vi "main(Test DQMH modules).vi"() -> ()   [LabVIEW 2018, in "Application.lvlib"] (continued)
                n6100 = To Variant(anything=T3."mux10_1_channel6" ("mux10_1(x6)_encode")) -> (Variant=w13208:variant)
                n6101 = To Variant(anything=T4."demux1_10_channel6" ("demux1_10(x6)_encode")) -> (Variant=w13204:variant)
                n6102 = To Variant(anything=bool[] [FALSE, FALSE, FALSE, TRUE, FALSE, FALSE]) -> (Variant=w13219:variant)
                n6103 = Bundle By Name(cluster=w13210, "command"="MEAS.AllRelaysOFF") -> (w13218:T9)
                n6104 = Bundle By Name(cluster=w13210, "command"="MEAS.mux10-1", "data"=w13208) -> (w13201:T9)
                n6105 = Bundle By Name(cluster=w13210, "command"="MEAS.demux1-10", "data"=w13204) -> (w13202:T9)
                n6106 = Bundle By Name(cluster=w13210, "command"="MEAS.eMIC", "data"=w13219) -> (w13203:T9)
                n6107 = Build Array(w13218, w13201, w13202, w13203) -> (w13196:T9[])
                n6108 = To Variant(anything=w13200) -> (Variant=w13199:variant)
                n6109 = To Variant(anything=w13200) -> (Variant=w13198:variant)
                n6110 = Bundle By Name(cluster=w13197, "command"="MEAS.requestAC", "data"=w13199) -> (w13216:T9)
                n6111 = Bundle By Name(cluster=w13197, "command"="Apps.WaitForEvent", "data"=w13198) -> (w13212:T9)
                n6112 = Bundle By Name(cluster=w13197, "command"="Apps.UI Update 1") -> (w13213:T9)
                n6113 = Bundle By Name(cluster=w13197, "command"="WaitFor") -> (w13195:T9)
                n6114 = Build Array (concatenate)(w13196, w13195, w13216, w13212, w13213) -> (w13211:T9[])
              }
              frame True {
                w13226 = T9 {"command"="", "data"=variant} ("element")
                w13248 = T9 {"command"="", "data"=variant} ("element")
                n6115 = To Variant(anything=T3."mux10_1_channel6" ("mux10_1(x6)_encode")) -> (Variant=w13255:variant)
                n6116 = To Variant(anything=T2."mux6_1_channel4_3" ("mux6_1(3wires)_encode")) -> (Variant=w13253:variant)
                n6117 = To Variant(anything=T4."demux1_10_channel6" ("demux1_10(x6)_encode")) -> (Variant=w13249:variant)
                n6118 = To Variant(anything=bool[] [FALSE, FALSE, FALSE, TRUE, FALSE, FALSE]) -> (Variant=w13245:variant)
                n6119 = Bundle By Name(cluster=w13248, "command"="MEAS.AllRelaysOFF") -> (w13244:T9)
                n6120 = Bundle By Name(cluster=w13248, "command"="MEAS.mux10-1", "data"=w13255) -> (w13243:T9)
                n6121 = Bundle By Name(cluster=w13248, "command"="MEAS.mux6_1", "data"=w13253) -> (w13242:T9)
                n6122 = Bundle By Name(cluster=w13248, "command"="MEAS.demux1-10", "data"=w13249) -> (w13241:T9)
                n6123 = Bundle By Name(cluster=w13248, "command"="MEAS.eMIC", "data"=w13245) -> (w13240:T9)
                n6124 = Build Array(w13244, w13243, w13242, w13241, w13240) -> (w13225:T9[])
                n6125 = To Variant(anything=w13230) -> (Variant=w13228:variant)
                n6126 = To Variant(anything=w13230) -> (Variant=w13227:variant)
                n6127 = Bundle By Name(cluster=w13226, "command"="WaitFor") -> (w13224:T9)
                n6128 = Bundle By Name(cluster=w13226, "command"="MEAS.DMM dual read") -> (w13237:T9)
                n6129 = Bundle By Name(cluster=w13226, "command"="MEAS.requestAC", "data"=w13228) -> (w13236:T9)
                n6130 = Bundle By Name(cluster=w13226, "command"="Apps.WaitForEvent", "data"=w13227) -> (w13231:T9)
                n6131 = Bundle By Name(cluster=w13226, "command"="Apps.UI Update 1") -> (w13232:T9)
                n6132 = Build Array (concatenate)(w13225, w13224, w13237, w13236, w13231, w13232) -> (w13229:T9[])
              }
            }
          }
          frame True {
            n6133 = Bundle By Name(cluster=T9 {"command"="", "data"=variant} ("element"), "command"="Apps.UI Update 1") -> (w13259:T9)
            n6134 = Build Array(w13259) -> (w13258:T9[])
          }
        }
        n6135 = for {
          tunnel: w13174 -> [w13269] mode=indexing
          tunnel: w13182 -> [w13270]
          tunnel: [w13266] -> w13184 mode=indexing
          n6136 = Unbundle By Name(w13269) -> ("command"=w13268:string, "data"=w13267:variant)
          n6137 = call "App enquece.vi"("command data"=w13267, "command"=w13268, "queue in"=w13270) -> ("error out"=w13266:errorcluster)  [unwired: 7 in, 1 out]
        }
        n6138 = Merge Errors(w13185, w13184) -> (w13183:errorcluster)
      }
      frame "Test DRV 35A" {
        w13274 = 35 ("DUT index(0-59)")
        n6139 = disable-structure shown="LOGGING==TRUE" {
          disable-tunnel: w13279 -> [w13362 _]
          frame condition #0 (active) {
            n6140 = Empty String/Path?(string/path=w13362) -> (empty?=w13364:bool)
            n6141 = Select(t="Quece timeout", s=w13364, f=w13362) -> (s? t:f=w13361:string)
            n6142 = call "string log (SubVI).vi"("state Name"=w13361) -> ()  [unwired: 9 in, 2 out]
          }
          frame condition #1 {
          }
        }
        n6143 = Flush Queue(queue=w13280) -> (queue out=w13281:refnum<queue>)  [unwired: 1 in, 2 out]
        n6144 = Decrement(x=w13274) -> (x-1=w13278:i32)
        n6145 = Index Array(array=w13275, index=w13278) -> (element=w13276:refnum<vi>)
        n6146 = call "FGV DRV stand.vi"() -> ("Sub-Test.DCV"=w13271:bool)  [unwired: 10 in, 1 out]
        n6147 = call "FGV Driver Data.vi"("DUT index(1-60)"=w13274) -> ("DUT SC"=w13272:bool)  [unwired: 7 in, 3 out]
        n6148 = property class="ColBox"(reference=w13276, "Value"=u32 10000536 ("DRV 1")) -> ()  [unwired: 1 in, 2 out]
        n6149 = case shown="False" w13272 {
          tunnel: w13274 -> [w13292 _]
          tunnel: [w13291 w13357] -> w13273
          tunnel: w13271 -> [w13290 _]
          frame False {
            n6150 = case shown="True" w13290 {
              tunnel: w13292 -> [w13299 w13329]
              tunnel: [w13310 w13328] -> w13291
              frame False {
                w13296 = T9 {"command"="", "data"=variant} ("element")
                w13309 = T9 {"command"="", "data"=variant} ("element")
                n6151 = To Variant(anything=T3."mux10_1_channel6" ("mux10_1(x6)_encode")) -> (Variant=w13307:variant)
                n6152 = To Variant(anything=T4."demux1_10_channel6" ("demux1_10(x6)_encode")) -> (Variant=w13303:variant)
                n6153 = To Variant(anything=bool[] [FALSE, FALSE, FALSE, FALSE, TRUE, FALSE]) -> (Variant=w13318:variant)
                n6154 = Bundle By Name(cluster=w13309, "command"="MEAS.AllRelaysOFF") -> (w13317:T9)
                n6155 = Bundle By Name(cluster=w13309, "command"="MEAS.mux10-1", "data"=w13307) -> (w13300:T9)
                n6156 = Bundle By Name(cluster=w13309, "command"="MEAS.demux1-10", "data"=w13303) -> (w13301:T9)
                n6157 = Bundle By Name(cluster=w13309, "command"="MEAS.eMIC", "data"=w13318) -> (w13302:T9)
                n6158 = Build Array(w13317, w13300, w13301, w13302) -> (w13295:T9[])
                n6159 = To Variant(anything=w13299) -> (Variant=w13298:variant)
                n6160 = To Variant(anything=w13299) -> (Variant=w13297:variant)
                n6161 = Bundle By Name(cluster=w13296, "command"="MEAS.requestAC", "data"=w13298) -> (w13315:T9)
                n6162 = Bundle By Name(cluster=w13296, "command"="Apps.WaitForEvent", "data"=w13297) -> (w13311:T9)
                n6163 = Bundle By Name(cluster=w13296, "command"="Apps.UI Update 1") -> (w13312:T9)
                n6164 = Bundle By Name(cluster=w13296, "command"="WaitFor") -> (w13294:T9)
                n6165 = Build Array (concatenate)(w13295, w13294, w13315, w13311, w13312) -> (w13310:T9[])
              }
              frame True {
                w13325 = T9 {"command"="", "data"=variant} ("element")
                w13347 = T9 {"command"="", "data"=variant} ("element")
                n6166 = To Variant(anything=T3."mux10_1_channel6" ("mux10_1(x6)_encode")) -> (Variant=w13354:variant)
                n6167 = To Variant(anything=T2."mux6_1_channel5_3" ("mux6_1(3wires)_encode")) -> (Variant=w13352:variant)
                n6168 = To Variant(anything=T4."demux1_10_channel6" ("demux1_10(x6)_encode")) -> (Variant=w13348:variant)
                n6169 = To Variant(anything=bool[] [FALSE, FALSE, FALSE, FALSE, TRUE, FALSE]) -> (Variant=w13344:variant)
                n6170 = Bundle By Name(cluster=w13347, "command"="MEAS.AllRelaysOFF") -> (w13343:T9)
                n6171 = Bundle By Name(cluster=w13347, "command"="MEAS.mux10-1", "data"=w13354) -> (w13342:T9)
                n6172 = Bundle By Name(cluster=w13347, "command"="MEAS.mux6_1", "data"=w13352) -> (w13341:T9)
                n6173 = Bundle By Name(cluster=w13347, "command"="MEAS.demux1-10", "data"=w13348) -> (w13340:T9)
                n6174 = Bundle By Name(cluster=w13347, "command"="MEAS.eMIC", "data"=w13344) -> (w13339:T9)
                n6175 = Build Array(w13343, w13342, w13341, w13340, w13339) -> (w13324:T9[])
                n6176 = To Variant(anything=w13329) -> (Variant=w13327:variant)
                n6177 = To Variant(anything=w13329) -> (Variant=w13326:variant)
                n6178 = Bundle By Name(cluster=w13325, "command"="WaitFor") -> (w13323:T9)
                n6179 = Bundle By Name(cluster=w13325, "command"="MEAS.DMM dual read") -> (w13336:T9)
                n6180 = Bundle By Name(cluster=w13325, "command"="MEAS.requestAC", "data"=w13327) -> (w13335:T9)
                n6181 = Bundle By Name(cluster=w13325, "command"="Apps.WaitForEvent", "data"=w13326) -> (w13330:T9)
                n6182 = Bundle By Name(cluster=w13325, "command"="Apps.UI Update 1") -> (w13331:T9)
                n6183 = Build Array (concatenate)(w13324, w13323, w13336, w13335, w13330, w13331) -> (w13328:T9[])
              }
            }
          }
          frame True {
            n6184 = Bundle By Name(cluster=T9 {"command"="", "data"=variant} ("element"), "command"="Apps.UI Update 1") -> (w13358:T9)
            n6185 = Build Array(w13358) -> (w13357:T9[])
          }
        }
        n6186 = for {
          tunnel: w13273 -> [w13368] mode=indexing
          tunnel: w13281 -> [w13369]
          tunnel: [w13365] -> w13283 mode=indexing
          n6187 = Unbundle By Name(w13368) -> ("command"=w13367:string, "data"=w13366:variant)
          n6188 = call "App enquece.vi"("command data"=w13366, "command"=w13367, "queue in"=w13369) -> ("error out"=w13365:errorcluster)  [unwired: 7 in, 1 out]
        }
        n6189 = Merge Errors(w13284, w13283) -> (w13282:errorcluster)
      }
      frame "Test DRV 36A" {
        w13373 = 36 ("DUT index(0-59)")
        n6190 = disable-structure shown="LOGGING==TRUE" {
          disable-tunnel: w13378 -> [w13461 _]
          frame condition #0 (active) {
            n6191 = Empty String/Path?(string/path=w13461) -> (empty?=w13463:bool)
            n6192 = Select(t="Quece timeout", s=w13463, f=w13461) -> (s? t:f=w13460:string)
            n6193 = call "string log (SubVI).vi"("state Name"=w13460) -> ()  [unwired: 9 in, 2 out]
          }
          frame condition #1 {
          }
        }
        n6194 = Flush Queue(queue=w13379) -> (queue out=w13380:refnum<queue>)  [unwired: 1 in, 2 out]
        n6195 = Decrement(x=w13373) -> (x-1=w13377:i32)
        n6196 = Index Array(array=w13374, index=w13377) -> (element=w13375:refnum<vi>)
        n6197 = call "FGV DRV stand.vi"() -> ("Sub-Test.DCV"=w13370:bool)  [unwired: 10 in, 1 out]
        n6198 = call "FGV Driver Data.vi"("DUT index(1-60)"=w13373) -> ("DUT SC"=w13371:bool)  [unwired: 7 in, 3 out]
        n6199 = property class="ColBox"(reference=w13375, "Value"=u32 10000536 ("DRV 1")) -> ()  [unwired: 1 in, 2 out]
        n6200 = case shown="False" w13371 {
          tunnel: w13373 -> [w13391 _]
          tunnel: [w13390 w13456] -> w13372
          tunnel: w13370 -> [w13389 _]
          frame False {
            n6201 = case shown="True" w13389 {
              tunnel: w13391 -> [w13398 w13428]
              tunnel: [w13409 w13427] -> w13390
              frame False {
                w13395 = T9 {"command"="", "data"=variant} ("element")
                w13408 = T9 {"command"="", "data"=variant} ("element")
                n6202 = To Variant(anything=T3."mux10_1_channel6" ("mux10_1(x6)_encode")) -> (Variant=w13406:variant)
                n6203 = To Variant(anything=T4."demux1_10_channel6" ("demux1_10(x6)_encode")) -> (Variant=w13402:variant)
                n6204 = To Variant(anything=bool[] [FALSE, FALSE, FALSE, FALSE, FALSE, TRUE]) -> (Variant=w13417:variant)
                n6205 = Bundle By Name(cluster=w13408, "command"="MEAS.AllRelaysOFF") -> (w13416:T9)
                n6206 = Bundle By Name(cluster=w13408, "command"="MEAS.mux10-1", "data"=w13406) -> (w13399:T9)
                n6207 = Bundle By Name(cluster=w13408, "command"="MEAS.demux1-10", "data"=w13402) -> (w13400:T9)
                n6208 = Bundle By Name(cluster=w13408, "command"="MEAS.eMIC", "data"=w13417) -> (w13401:T9)
                n6209 = Build Array(w13416, w13399, w13400, w13401) -> (w13394:T9[])
                n6210 = To Variant(anything=w13398) -> (Variant=w13397:variant)
                n6211 = To Variant(anything=w13398) -> (Variant=w13396:variant)
                n6212 = Bundle By Name(cluster=w13395, "command"="MEAS.requestAC", "data"=w13397) -> (w13414:T9)
                n6213 = Bundle By Name(cluster=w13395, "command"="Apps.WaitForEvent", "data"=w13396) -> (w13410:T9)
                n6214 = Bundle By Name(cluster=w13395, "command"="Apps.UI Update 1") -> (w13411:T9)
                n6215 = Bundle By Name(cluster=w13395, "command"="WaitFor") -> (w13393:T9)
                n6216 = Build Array (concatenate)(w13394, w13393, w13414, w13410, w13411) -> (w13409:T9[])
              }
              frame True {
                w13424 = T9 {"command"="", "data"=variant} ("element")
                w13446 = T9 {"command"="", "data"=variant} ("element")
                n6217 = To Variant(anything=T3."mux10_1_channel6" ("mux10_1(x6)_encode")) -> (Variant=w13453:variant)
                n6218 = To Variant(anything=T2."mux6_1_channel6_3" ("mux6_1(3wires)_encode")) -> (Variant=w13451:variant)
                n6219 = To Variant(anything=T4."demux1_10_channel6" ("demux1_10(x6)_encode")) -> (Variant=w13447:variant)
                n6220 = To Variant(anything=bool[] [FALSE, FALSE, FALSE, FALSE, FALSE, TRUE]) -> (Variant=w13443:variant)
                n6221 = Bundle By Name(cluster=w13446, "command"="MEAS.AllRelaysOFF") -> (w13442:T9)
                n6222 = Bundle By Name(cluster=w13446, "command"="MEAS.mux10-1", "data"=w13453) -> (w13441:T9)
                n6223 = Bundle By Name(cluster=w13446, "command"="MEAS.mux6_1", "data"=w13451) -> (w13440:T9)
                n6224 = Bundle By Name(cluster=w13446, "command"="MEAS.demux1-10", "data"=w13447) -> (w13439:T9)
                n6225 = Bundle By Name(cluster=w13446, "command"="MEAS.eMIC", "data"=w13443) -> (w13438:T9)
                n6226 = Build Array(w13442, w13441, w13440, w13439, w13438) -> (w13423:T9[])
                n6227 = To Variant(anything=w13428) -> (Variant=w13426:variant)
                n6228 = To Variant(anything=w13428) -> (Variant=w13425:variant)
                n6229 = Bundle By Name(cluster=w13424, "command"="WaitFor") -> (w13422:T9)
                n6230 = Bundle By Name(cluster=w13424, "command"="MEAS.DMM dual read") -> (w13435:T9)
                n6231 = Bundle By Name(cluster=w13424, "command"="MEAS.requestAC", "data"=w13426) -> (w13434:T9)
                n6232 = Bundle By Name(cluster=w13424, "command"="Apps.WaitForEvent", "data"=w13425) -> (w13429:T9)
                n6233 = Bundle By Name(cluster=w13424, "command"="Apps.UI Update 1") -> (w13430:T9)
                n6234 = Build Array (concatenate)(w13423, w13422, w13435, w13434, w13429, w13430) -> (w13427:T9[])
              }
            }
          }
          frame True {
            n6235 = Bundle By Name(cluster=T9 {"command"="", "data"=variant} ("element"), "command"="Apps.UI Update 1") -> (w13457:T9)
            n6236 = Build Array(w13457) -> (w13456:T9[])
          }
        }
        n6237 = for {
          tunnel: w13372 -> [w13467] mode=indexing
          tunnel: w13380 -> [w13468]
          tunnel: [w13464] -> w13382 mode=indexing
          n6238 = Unbundle By Name(w13467) -> ("command"=w13466:string, "data"=w13465:variant)
          n6239 = call "App enquece.vi"("command data"=w13465, "command"=w13466, "queue in"=w13468) -> ("error out"=w13464:errorcluster)  [unwired: 7 in, 1 out]
        }
        n6240 = Merge Errors(w13383, w13382) -> (w13381:errorcluster)
      }
      frame "Test DRV 37A" {
        w13472 = 37 ("DUT index(0-59)")
        n6241 = disable-structure shown="LOGGING==TRUE" {
          disable-tunnel: w13477 -> [w13560 _]
          frame condition #0 (active) {
            n6242 = Empty String/Path?(string/path=w13560) -> (empty?=w13562:bool)
            n6243 = Select(t="Quece timeout", s=w13562, f=w13560) -> (s? t:f=w13559:string)
            n6244 = call "string log (SubVI).vi"("state Name"=w13559) -> ()  [unwired: 9 in, 2 out]
          }
          frame condition #1 {
          }
        }
        n6245 = Flush Queue(queue=w13478) -> (queue out=w13479:refnum<queue>)  [unwired: 1 in, 2 out]
        n6246 = Decrement(x=w13472) -> (x-1=w13476:i32)
        n6247 = Index Array(array=w13473, index=w13476) -> (element=w13474:refnum<vi>)
        n6248 = call "FGV DRV stand.vi"() -> ("Sub-Test.DCV"=w13469:bool)  [unwired: 10 in, 1 out]
        n6249 = call "FGV Driver Data.vi"("DUT index(1-60)"=w13472) -> ("DUT SC"=w13470:bool)  [unwired: 7 in, 3 out]
        n6250 = property class="ColBox"(reference=w13474, "Value"=u32 10000536 ("DRV 1")) -> ()  [unwired: 1 in, 2 out]
        n6251 = case shown="False" w13470 {
          tunnel: w13472 -> [w13490 _]
          tunnel: [w13489 w13555] -> w13471
          tunnel: w13469 -> [w13488 _]
          frame False {
            n6252 = case shown="False" w13488 {
              tunnel: w13490 -> [w13497 w13527]
              tunnel: [w13508 w13526] -> w13489
              frame False {
                w13494 = T9 {"command"="", "data"=variant} ("element")
                w13507 = T9 {"command"="", "data"=variant} ("element")
                n6253 = To Variant(anything=T3."mux10_1_channel7" ("mux10_1(x6)_encode")) -> (Variant=w13505:variant)
                n6254 = To Variant(anything=T4."demux1_10_channel7" ("demux1_10(x6)_encode")) -> (Variant=w13501:variant)
                n6255 = To Variant(anything=bool[] [TRUE, FALSE, FALSE, FALSE, FALSE, FALSE]) -> (Variant=w13516:variant)
                n6256 = Bundle By Name(cluster=w13507, "command"="MEAS.AllRelaysOFF") -> (w13515:T9)
                n6257 = Bundle By Name(cluster=w13507, "command"="MEAS.mux10-1", "data"=w13505) -> (w13498:T9)
                n6258 = Bundle By Name(cluster=w13507, "command"="MEAS.demux1-10", "data"=w13501) -> (w13499:T9)
                n6259 = Bundle By Name(cluster=w13507, "command"="MEAS.eMIC", "data"=w13516) -> (w13500:T9)
                n6260 = Build Array(w13515, w13498, w13499, w13500) -> (w13493:T9[])
                n6261 = To Variant(anything=w13497) -> (Variant=w13496:variant)
                n6262 = To Variant(anything=w13497) -> (Variant=w13495:variant)
                n6263 = Bundle By Name(cluster=w13494, "command"="MEAS.requestAC", "data"=w13496) -> (w13513:T9)
                n6264 = Bundle By Name(cluster=w13494, "command"="Apps.WaitForEvent", "data"=w13495) -> (w13509:T9)
                n6265 = Bundle By Name(cluster=w13494, "command"="Apps.UI Update 1") -> (w13510:T9)
                n6266 = Bundle By Name(cluster=w13494, "command"="WaitFor") -> (w13492:T9)
                n6267 = Build Array (concatenate)(w13493, w13492, w13513, w13509, w13510) -> (w13508:T9[])
              }
              frame True {
                w13523 = T9 {"command"="", "data"=variant} ("element")
                w13545 = T9 {"command"="", "data"=variant} ("element")
                n6268 = To Variant(anything=T3."mux10_1_channel7" ("mux10_1(x6)_encode")) -> (Variant=w13552:variant)
                n6269 = To Variant(anything=T2."mux6_1_channel1_3" ("mux6_1(3wires)_encode")) -> (Variant=w13550:variant)
                n6270 = To Variant(anything=T4."demux1_10_channel7" ("demux1_10(x6)_encode")) -> (Variant=w13546:variant)
                n6271 = To Variant(anything=bool[] [TRUE, FALSE, FALSE, FALSE, FALSE, FALSE]) -> (Variant=w13542:variant)
                n6272 = Bundle By Name(cluster=w13545, "command"="MEAS.AllRelaysOFF") -> (w13541:T9)
                n6273 = Bundle By Name(cluster=w13545, "command"="MEAS.mux10-1", "data"=w13552) -> (w13540:T9)
                n6274 = Bundle By Name(cluster=w13545, "command"="MEAS.mux6_1", "data"=w13550) -> (w13539:T9)
                n6275 = Bundle By Name(cluster=w13545, "command"="MEAS.demux1-10", "data"=w13546) -> (w13538:T9)
                n6276 = Bundle By Name(cluster=w13545, "command"="MEAS.eMIC", "data"=w13542) -> (w13537:T9)
                n6277 = Build Array(w13541, w13540, w13539, w13538, w13537) -> (w13522:T9[])
                n6278 = To Variant(anything=w13527) -> (Variant=w13525:variant)
                n6279 = To Variant(anything=w13527) -> (Variant=w13524:variant)
                n6280 = Bundle By Name(cluster=w13523, "command"="WaitFor") -> (w13521:T9)
                n6281 = Bundle By Name(cluster=w13523, "command"="MEAS.DMM dual read") -> (w13534:T9)
                n6282 = Bundle By Name(cluster=w13523, "command"="MEAS.requestAC", "data"=w13525) -> (w13533:T9)
                n6283 = Bundle By Name(cluster=w13523, "command"="Apps.WaitForEvent", "data"=w13524) -> (w13528:T9)
                n6284 = Bundle By Name(cluster=w13523, "command"="Apps.UI Update 1") -> (w13529:T9)
                n6285 = Build Array (concatenate)(w13522, w13521, w13534, w13533, w13528, w13529) -> (w13526:T9[])
              }
            }
          }
          frame True {
            n6286 = Bundle By Name(cluster=T9 {"command"="", "data"=variant} ("element"), "command"="Apps.UI Update 1") -> (w13556:T9)
            n6287 = Build Array(w13556) -> (w13555:T9[])
          }
        }
        n6288 = for {
          tunnel: w13471 -> [w13566] mode=indexing
          tunnel: w13479 -> [w13567]
          tunnel: [w13563] -> w13481 mode=indexing
          n6289 = Unbundle By Name(w13566) -> ("command"=w13565:string, "data"=w13564:variant)
          n6290 = call "App enquece.vi"("command data"=w13564, "command"=w13565, "queue in"=w13567) -> ("error out"=w13563:errorcluster)  [unwired: 7 in, 1 out]
        }
        n6291 = Merge Errors(w13482, w13481) -> (w13480:errorcluster)
      }
      frame "Test DRV 38A" {
        w13571 = 38 ("DUT index(0-59)")
        n6292 = disable-structure shown="LOGGING==TRUE" {
          disable-tunnel: w13576 -> [w13659 _]
          frame condition #0 (active) {
            n6293 = Empty String/Path?(string/path=w13659) -> (empty?=w13661:bool)
            n6294 = Select(t="Quece timeout", s=w13661, f=w13659) -> (s? t:f=w13658:string)
            n6295 = call "string log (SubVI).vi"("state Name"=w13658) -> ()  [unwired: 9 in, 2 out]
          }
          frame condition #1 {
          }
        }
        n6296 = Flush Queue(queue=w13577) -> (queue out=w13578:refnum<queue>)  [unwired: 1 in, 2 out]
        n6297 = Decrement(x=w13571) -> (x-1=w13575:i32)
        n6298 = Index Array(array=w13572, index=w13575) -> (element=w13573:refnum<vi>)
        n6299 = call "FGV DRV stand.vi"() -> ("Sub-Test.DCV"=w13568:bool)  [unwired: 10 in, 1 out]
        n6300 = call "FGV Driver Data.vi"("DUT index(1-60)"=w13571) -> ("DUT SC"=w13569:bool)  [unwired: 7 in, 3 out]
        n6301 = property class="ColBox"(reference=w13573, "Value"=u32 10000536 ("DRV 1")) -> ()  [unwired: 1 in, 2 out]
        n6302 = case shown="False" w13569 {
          tunnel: w13571 -> [w13589 _]
          tunnel: [w13588 w13654] -> w13570
          tunnel: w13568 -> [w13587 _]
          frame False {
            n6303 = case shown="True" w13587 {
              tunnel: w13589 -> [w13596 w13626]
              tunnel: [w13607 w13625] -> w13588
              frame False {
                w13593 = T9 {"command"="", "data"=variant} ("element")
                w13606 = T9 {"command"="", "data"=variant} ("element")
                n6304 = To Variant(anything=T3."mux10_1_channel7" ("mux10_1(x6)_encode")) -> (Variant=w13604:variant)
                n6305 = To Variant(anything=T4."demux1_10_channel7" ("demux1_10(x6)_encode")) -> (Variant=w13600:variant)
                n6306 = To Variant(anything=bool[] [FALSE, TRUE, FALSE, FALSE, FALSE, FALSE]) -> (Variant=w13615:variant)
                n6307 = Bundle By Name(cluster=w13606, "command"="MEAS.AllRelaysOFF") -> (w13614:T9)
                n6308 = Bundle By Name(cluster=w13606, "command"="MEAS.mux10-1", "data"=w13604) -> (w13597:T9)
                n6309 = Bundle By Name(cluster=w13606, "command"="MEAS.demux1-10", "data"=w13600) -> (w13598:T9)
                n6310 = Bundle By Name(cluster=w13606, "command"="MEAS.eMIC", "data"=w13615) -> (w13599:T9)
                n6311 = Build Array(w13614, w13597, w13598, w13599) -> (w13592:T9[])
                n6312 = To Variant(anything=w13596) -> (Variant=w13595:variant)
                n6313 = To Variant(anything=w13596) -> (Variant=w13594:variant)
                n6314 = Bundle By Name(cluster=w13593, "command"="MEAS.requestAC", "data"=w13595) -> (w13612:T9)
                n6315 = Bundle By Name(cluster=w13593, "command"="Apps.WaitForEvent", "data"=w13594) -> (w13608:T9)
                n6316 = Bundle By Name(cluster=w13593, "command"="Apps.UI Update 1") -> (w13609:T9)
                n6317 = Bundle By Name(cluster=w13593, "command"="WaitFor") -> (w13591:T9)
                n6318 = Build Array (concatenate)(w13592, w13591, w13612, w13608, w13609) -> (w13607:T9[])
              }
              frame True {
                w13622 = T9 {"command"="", "data"=variant} ("element")
                w13644 = T9 {"command"="", "data"=variant} ("element")
                n6319 = To Variant(anything=T3."mux10_1_channel7" ("mux10_1(x6)_encode")) -> (Variant=w13651:variant)
                n6320 = To Variant(anything=T2."mux6_1_channel2_3" ("mux6_1(3wires)_encode")) -> (Variant=w13649:variant)
                n6321 = To Variant(anything=T4."demux1_10_channel7" ("demux1_10(x6)_encode")) -> (Variant=w13645:variant)
                n6322 = To Variant(anything=bool[] [FALSE, TRUE, FALSE, FALSE, FALSE, FALSE]) -> (Variant=w13641:variant)
                n6323 = Bundle By Name(cluster=w13644, "command"="MEAS.AllRelaysOFF") -> (w13640:T9)
                n6324 = Bundle By Name(cluster=w13644, "command"="MEAS.mux10-1", "data"=w13651) -> (w13639:T9)
                n6325 = Bundle By Name(cluster=w13644, "command"="MEAS.mux6_1", "data"=w13649) -> (w13638:T9)
                n6326 = Bundle By Name(cluster=w13644, "command"="MEAS.demux1-10", "data"=w13645) -> (w13637:T9)
                n6327 = Bundle By Name(cluster=w13644, "command"="MEAS.eMIC", "data"=w13641) -> (w13636:T9)
                n6328 = Build Array(w13640, w13639, w13638, w13637, w13636) -> (w13621:T9[])
                n6329 = To Variant(anything=w13626) -> (Variant=w13624:variant)
                n6330 = To Variant(anything=w13626) -> (Variant=w13623:variant)
                n6331 = Bundle By Name(cluster=w13622, "command"="WaitFor") -> (w13620:T9)
                n6332 = Bundle By Name(cluster=w13622, "command"="MEAS.DMM dual read") -> (w13633:T9)
                n6333 = Bundle By Name(cluster=w13622, "command"="MEAS.requestAC", "data"=w13624) -> (w13632:T9)
                n6334 = Bundle By Name(cluster=w13622, "command"="Apps.WaitForEvent", "data"=w13623) -> (w13627:T9)
                n6335 = Bundle By Name(cluster=w13622, "command"="Apps.UI Update 1") -> (w13628:T9)
                n6336 = Build Array (concatenate)(w13621, w13620, w13633, w13632, w13627, w13628) -> (w13625:T9[])
              }
            }
          }
          frame True {
            n6337 = Bundle By Name(cluster=T9 {"command"="", "data"=variant} ("element"), "command"="Apps.UI Update 1") -> (w13655:T9)
            n6338 = Build Array(w13655) -> (w13654:T9[])
          }
        }
        n6339 = for {
          tunnel: w13570 -> [w13665] mode=indexing
          tunnel: w13578 -> [w13666]
          tunnel: [w13662] -> w13580 mode=indexing
          n6340 = Unbundle By Name(w13665) -> ("command"=w13664:string, "data"=w13663:variant)
          n6341 = call "App enquece.vi"("command data"=w13663, "command"=w13664, "queue in"=w13666) -> ("error out"=w13662:errorcluster)  [unwired: 7 in, 1 out]
        }
        n6342 = Merge Errors(w13581, w13580) -> (w13579:errorcluster)
      }
      frame "Test DRV 39A" {
        w13670 = 39 ("DUT index(0-59)")
        n6343 = disable-structure shown="LOGGING==TRUE" {
          disable-tunnel: w13675 -> [w13758 _]
          frame condition #0 (active) {
            n6344 = Empty String/Path?(string/path=w13758) -> (empty?=w13760:bool)
            n6345 = Select(t="Quece timeout", s=w13760, f=w13758) -> (s? t:f=w13757:string)
            n6346 = call "string log (SubVI).vi"("state Name"=w13757) -> ()  [unwired: 9 in, 2 out]
          }
          frame condition #1 {
          }
        }
        n6347 = Flush Queue(queue=w13676) -> (queue out=w13677:refnum<queue>)  [unwired: 1 in, 2 out]
        n6348 = Decrement(x=w13670) -> (x-1=w13674:i32)
        n6349 = Index Array(array=w13671, index=w13674) -> (element=w13672:refnum<vi>)
        n6350 = call "FGV DRV stand.vi"() -> ("Sub-Test.DCV"=w13667:bool)  [unwired: 10 in, 1 out]
        n6351 = call "FGV Driver Data.vi"("DUT index(1-60)"=w13670) -> ("DUT SC"=w13668:bool)  [unwired: 7 in, 3 out]
        n6352 = property class="ColBox"(reference=w13672, "Value"=u32 10000536 ("DRV 1")) -> ()  [unwired: 1 in, 2 out]
        n6353 = case shown="False" w13668 {
          tunnel: w13670 -> [w13688 _]
          tunnel: [w13687 w13753] -> w13669
          tunnel: w13667 -> [w13686 _]
          frame False {
            n6354 = case shown="False" w13686 {
              tunnel: w13688 -> [w13695 w13725]
              tunnel: [w13706 w13724] -> w13687
              frame False {
                w13692 = T9 {"command"="", "data"=variant} ("element")
                w13705 = T9 {"command"="", "data"=variant} ("element")
                n6355 = To Variant(anything=T3."mux10_1_channel7" ("mux10_1(x6)_encode")) -> (Variant=w13703:variant)
                n6356 = To Variant(anything=T4."demux1_10_channel7" ("demux1_10(x6)_encode")) -> (Variant=w13699:variant)
                n6357 = To Variant(anything=bool[] [FALSE, FALSE, TRUE, FALSE, FALSE, FALSE]) -> (Variant=w13714:variant)
                n6358 = Bundle By Name(cluster=w13705, "command"="MEAS.AllRelaysOFF") -> (w13713:T9)
                n6359 = Bundle By Name(cluster=w13705, "command"="MEAS.mux10-1", "data"=w13703) -> (w13696:T9)
                n6360 = Bundle By Name(cluster=w13705, "command"="MEAS.demux1-10", "data"=w13699) -> (w13697:T9)
                n6361 = Bundle By Name(cluster=w13705, "command"="MEAS.eMIC", "data"=w13714) -> (w13698:T9)
                n6362 = Build Array(w13713, w13696, w13697, w13698) -> (w13691:T9[])
                n6363 = To Variant(anything=w13695) -> (Variant=w13694:variant)
                n6364 = To Variant(anything=w13695) -> (Variant=w13693:variant)
                n6365 = Bundle By Name(cluster=w13692, "command"="MEAS.requestAC", "data"=w13694) -> (w13711:T9)
                n6366 = Bundle By Name(cluster=w13692, "command"="Apps.WaitForEvent", "data"=w13693) -> (w13707:T9)
                n6367 = Bundle By Name(cluster=w13692, "command"="Apps.UI Update 1") -> (w13708:T9)
                n6368 = Bundle By Name(cluster=w13692, "command"="WaitFor") -> (w13690:T9)
                n6369 = Build Array (concatenate)(w13691, w13690, w13711, w13707, w13708) -> (w13706:T9[])
              }
              frame True {
                w13721 = T9 {"command"="", "data"=variant} ("element")
                w13743 = T9 {"command"="", "data"=variant} ("element")
                n6370 = To Variant(anything=T3."mux10_1_channel7" ("mux10_1(x6)_encode")) -> (Variant=w13750:variant)
                n6371 = To Variant(anything=T2."mux6_1_channel3_3" ("mux6_1(3wires)_encode")) -> (Variant=w13748:variant)
                n6372 = To Variant(anything=T4."demux1_10_channel7" ("demux1_10(x6)_encode")) -> (Variant=w13744:variant)
                n6373 = To Variant(anything=bool[] [FALSE, FALSE, TRUE, FALSE, FALSE, FALSE]) -> (Variant=w13740:variant)
                n6374 = Bundle By Name(cluster=w13743, "command"="MEAS.AllRelaysOFF") -> (w13739:T9)
                n6375 = Bundle By Name(cluster=w13743, "command"="MEAS.mux10-1", "data"=w13750) -> (w13738:T9)
                n6376 = Bundle By Name(cluster=w13743, "command"="MEAS.mux6_1", "data"=w13748) -> (w13737:T9)
                n6377 = Bundle By Name(cluster=w13743, "command"="MEAS.demux1-10", "data"=w13744) -> (w13736:T9)
                n6378 = Bundle By Name(cluster=w13743, "command"="MEAS.eMIC", "data"=w13740) -> (w13735:T9)
                n6379 = Build Array(w13739, w13738, w13737, w13736, w13735) -> (w13720:T9[])
                n6380 = To Variant(anything=w13725) -> (Variant=w13723:variant)
                n6381 = To Variant(anything=w13725) -> (Variant=w13722:variant)
                n6382 = Bundle By Name(cluster=w13721, "command"="WaitFor") -> (w13719:T9)
                n6383 = Bundle By Name(cluster=w13721, "command"="MEAS.DMM dual read") -> (w13732:T9)
                n6384 = Bundle By Name(cluster=w13721, "command"="MEAS.requestAC", "data"=w13723) -> (w13731:T9)
                n6385 = Bundle By Name(cluster=w13721, "command"="Apps.WaitForEvent", "data"=w13722) -> (w13726:T9)
                n6386 = Bundle By Name(cluster=w13721, "command"="Apps.UI Update 1") -> (w13727:T9)
                n6387 = Build Array (concatenate)(w13720, w13719, w13732, w13731, w13726, w13727) -> (w13724:T9[])
              }
            }
          }
          frame True {
            n6388 = Bundle By Name(cluster=T9 {"command"="", "data"=variant} ("element"), "command"="Apps.UI Update 1") -> (w13754:T9)
            n6389 = Build Array(w13754) -> (w13753:T9[])
          }
        }
        n6390 = for {
          tunnel: w13669 -> [w13764] mode=indexing
          tunnel: w13677 -> [w13765]
          tunnel: [w13761] -> w13679 mode=indexing
          n6391 = Unbundle By Name(w13764) -> ("command"=w13763:string, "data"=w13762:variant)
          n6392 = call "App enquece.vi"("command data"=w13762, "command"=w13763, "queue in"=w13765) -> ("error out"=w13761:errorcluster)  [unwired: 7 in, 1 out]
        }
        n6393 = Merge Errors(w13680, w13679) -> (w13678:errorcluster)
      }
      frame "Test DRV 40A" {
        w13769 = 40 ("DUT index(0-59)")
        n6394 = disable-structure shown="LOGGING==TRUE" {
          disable-tunnel: w13774 -> [w13857 _]
          frame condition #0 (active) {
            n6395 = Empty String/Path?(string/path=w13857) -> (empty?=w13859:bool)
            n6396 = Select(t="Quece timeout", s=w13859, f=w13857) -> (s? t:f=w13856:string)
            n6397 = call "string log (SubVI).vi"("state Name"=w13856) -> ()  [unwired: 9 in, 2 out]
          }
          frame condition #1 {
          }
        }
        n6398 = Flush Queue(queue=w13775) -> (queue out=w13776:refnum<queue>)  [unwired: 1 in, 2 out]
        n6399 = Decrement(x=w13769) -> (x-1=w13773:i32)
        n6400 = Index Array(array=w13770, index=w13773) -> (element=w13771:refnum<vi>)
        n6401 = call "FGV DRV stand.vi"() -> ("Sub-Test.DCV"=w13766:bool)  [unwired: 10 in, 1 out]
        n6402 = call "FGV Driver Data.vi"("DUT index(1-60)"=w13769) -> ("DUT SC"=w13767:bool)  [unwired: 7 in, 3 out]
        n6403 = property class="ColBox"(reference=w13771, "Value"=u32 10000536 ("DRV 1")) -> ()  [unwired: 1 in, 2 out]
        n6404 = case shown="False" w13767 {
          tunnel: w13769 -> [w13787 _]
          tunnel: [w13786 w13852] -> w13768
          tunnel: w13766 -> [w13785 _]
          frame False {
            n6405 = case shown="True" w13785 {
              tunnel: w13787 -> [w13794 w13824]
              tunnel: [w13805 w13823] -> w13786
              frame False {
                w13791 = T9 {"command"="", "data"=variant} ("element")
                w13804 = T9 {"command"="", "data"=variant} ("element")
                n6406 = To Variant(anything=T3."mux10_1_channel7" ("mux10_1(x6)_encode")) -> (Variant=w13802:variant)
                n6407 = To Variant(anything=T4."demux1_10_channel7" ("demux1_10(x6)_encode")) -> (Variant=w13798:variant)
                n6408 = To Variant(anything=bool[] [FALSE, FALSE, FALSE, TRUE, FALSE, FALSE]) -> (Variant=w13813:variant)
                n6409 = Bundle By Name(cluster=w13804, "command"="MEAS.AllRelaysOFF") -> (w13812:T9)
                n6410 = Bundle By Name(cluster=w13804, "command"="MEAS.mux10-1", "data"=w13802) -> (w13795:T9)
                n6411 = Bundle By Name(cluster=w13804, "command"="MEAS.demux1-10", "data"=w13798) -> (w13796:T9)
                n6412 = Bundle By Name(cluster=w13804, "command"="MEAS.eMIC", "data"=w13813) -> (w13797:T9)
                n6413 = Build Array(w13812, w13795, w13796, w13797) -> (w13790:T9[])
                n6414 = To Variant(anything=w13794) -> (Variant=w13793:variant)
                n6415 = To Variant(anything=w13794) -> (Variant=w13792:variant)
                n6416 = Bundle By Name(cluster=w13791, "command"="MEAS.requestAC", "data"=w13793) -> (w13810:T9)
                n6417 = Bundle By Name(cluster=w13791, "command"="Apps.WaitForEvent", "data"=w13792) -> (w13806:T9)
                n6418 = Bundle By Name(cluster=w13791, "command"="Apps.UI Update 1") -> (w13807:T9)
                n6419 = Bundle By Name(cluster=w13791, "command"="WaitFor") -> (w13789:T9)
                n6420 = Build Array (concatenate)(w13790, w13789, w13810, w13806, w13807) -> (w13805:T9[])
              }
              frame True {
                w13820 = T9 {"command"="", "data"=variant} ("element")
                w13842 = T9 {"command"="", "data"=variant} ("element")
                n6421 = To Variant(anything=T3."mux10_1_channel7" ("mux10_1(x6)_encode")) -> (Variant=w13849:variant)
                n6422 = To Variant(anything=T2."mux6_1_channel4_3" ("mux6_1(3wires)_encode")) -> (Variant=w13847:variant)
                n6423 = To Variant(anything=T4."demux1_10_channel7" ("demux1_10(x6)_encode")) -> (Variant=w13843:variant)
                n6424 = To Variant(anything=bool[] [FALSE, FALSE, FALSE, TRUE, FALSE, FALSE]) -> (Variant=w13839:variant)
                n6425 = Bundle By Name(cluster=w13842, "command"="MEAS.AllRelaysOFF") -> (w13838:T9)
                n6426 = Bundle By Name(cluster=w13842, "command"="MEAS.mux10-1", "data"=w13849) -> (w13837:T9)
                n6427 = Bundle By Name(cluster=w13842, "command"="MEAS.mux6_1", "data"=w13847) -> (w13836:T9)
                n6428 = Bundle By Name(cluster=w13842, "command"="MEAS.demux1-10", "data"=w13843) -> (w13835:T9)
                n6429 = Bundle By Name(cluster=w13842, "command"="MEAS.eMIC", "data"=w13839) -> (w13834:T9)
                n6430 = Build Array(w13838, w13837, w13836, w13835, w13834) -> (w13819:T9[])
                n6431 = To Variant(anything=w13824) -> (Variant=w13822:variant)
                n6432 = To Variant(anything=w13824) -> (Variant=w13821:variant)
                n6433 = Bundle By Name(cluster=w13820, "command"="WaitFor") -> (w13818:T9)
                n6434 = Bundle By Name(cluster=w13820, "command"="MEAS.DMM dual read") -> (w13831:T9)
                n6435 = Bundle By Name(cluster=w13820, "command"="MEAS.requestAC", "data"=w13822) -> (w13830:T9)
                n6436 = Bundle By Name(cluster=w13820, "command"="Apps.WaitForEvent", "data"=w13821) -> (w13825:T9)
                n6437 = Bundle By Name(cluster=w13820, "command"="Apps.UI Update 1") -> (w13826:T9)
                n6438 = Build Array (concatenate)(w13819, w13818, w13831, w13830, w13825, w13826) -> (w13823:T9[])
              }
            }
          }
          frame True {
            n6439 = Bundle By Name(cluster=T9 {"command"="", "data"=variant} ("element"), "command"="Apps.UI Update 1") -> (w13853:T9)
            n6440 = Build Array(w13853) -> (w13852:T9[])
          }
        }
        n6441 = for {
          tunnel: w13768 -> [w13863] mode=indexing
          tunnel: w13776 -> [w13864]
          tunnel: [w13860] -> w13778 mode=indexing
          n6442 = Unbundle By Name(w13863) -> ("command"=w13862:string, "data"=w13861:variant)
          n6443 = call "App enquece.vi"("command data"=w13861, "command"=w13862, "queue in"=w13864) -> ("error out"=w13860:errorcluster)  [unwired: 7 in, 1 out]
        }
        n6444 = Merge Errors(w13779, w13778) -> (w13777:errorcluster)
      }
      frame "Test DRV 41A" {
        w13868 = 41 ("DUT index(0-59)")
        n6445 = disable-structure shown="LOGGING==TRUE" {
          disable-tunnel: w13873 -> [w13956 _]
          frame condition #0 (active) {
            n6446 = Empty String/Path?(string/path=w13956) -> (empty?=w13958:bool)
            n6447 = Select(t="Quece timeout", s=w13958, f=w13956) -> (s? t:f=w13955:string)
            n6448 = call "string log (SubVI).vi"("state Name"=w13955) -> ()  [unwired: 9 in, 2 out]
          }
          frame condition #1 {
          }
        }
        n6449 = Flush Queue(queue=w13874) -> (queue out=w13875:refnum<queue>)  [unwired: 1 in, 2 out]
        n6450 = Decrement(x=w13868) -> (x-1=w13872:i32)
        n6451 = Index Array(array=w13869, index=w13872) -> (element=w13870:refnum<vi>)
        n6452 = call "FGV DRV stand.vi"() -> ("Sub-Test.DCV"=w13865:bool)  [unwired: 10 in, 1 out]
        n6453 = call "FGV Driver Data.vi"("DUT index(1-60)"=w13868) -> ("DUT SC"=w13866:bool)  [unwired: 7 in, 3 out]
        n6454 = property class="ColBox"(reference=w13870, "Value"=u32 10000536 ("DRV 1")) -> ()  [unwired: 1 in, 2 out]
        n6455 = case shown="False" w13866 {
          tunnel: w13868 -> [w13886 _]
          tunnel: [w13885 w13951] -> w13867
          tunnel: w13865 -> [w13884 _]
          frame False {
            n6456 = case shown="False" w13884 {
              tunnel: w13886 -> [w13893 w13923]
              tunnel: [w13904 w13922] -> w13885
              frame False {
                w13890 = T9 {"command"="", "data"=variant} ("element")
                w13903 = T9 {"command"="", "data"=variant} ("element")
                n6457 = To Variant(anything=T3."mux10_1_channel7" ("mux10_1(x6)_encode")) -> (Variant=w13901:variant)
                n6458 = To Variant(anything=T4."demux1_10_channel7" ("demux1_10(x6)_encode")) -> (Variant=w13897:variant)
                n6459 = To Variant(anything=bool[] [FALSE, FALSE, FALSE, FALSE, TRUE, FALSE]) -> (Variant=w13912:variant)
                n6460 = Bundle By Name(cluster=w13903, "command"="MEAS.AllRelaysOFF") -> (w13911:T9)
                n6461 = Bundle By Name(cluster=w13903, "command"="MEAS.mux10-1", "data"=w13901) -> (w13894:T9)
                n6462 = Bundle By Name(cluster=w13903, "command"="MEAS.demux1-10", "data"=w13897) -> (w13895:T9)
                n6463 = Bundle By Name(cluster=w13903, "command"="MEAS.eMIC", "data"=w13912) -> (w13896:T9)
                n6464 = Build Array(w13911, w13894, w13895, w13896) -> (w13889:T9[])
                n6465 = To Variant(anything=w13893) -> (Variant=w13892:variant)
                n6466 = To Variant(anything=w13893) -> (Variant=w13891:variant)
                n6467 = Bundle By Name(cluster=w13890, "command"="MEAS.requestAC", "data"=w13892) -> (w13909:T9)
                n6468 = Bundle By Name(cluster=w13890, "command"="Apps.WaitForEvent", "data"=w13891) -> (w13905:T9)
                n6469 = Bundle By Name(cluster=w13890, "command"="Apps.UI Update 1") -> (w13906:T9)
                n6470 = Bundle By Name(cluster=w13890, "command"="WaitFor") -> (w13888:T9)
                n6471 = Build Array (concatenate)(w13889, w13888, w13909, w13905, w13906) -> (w13904:T9[])
              }
              frame True {
                w13919 = T9 {"command"="", "data"=variant} ("element")
                w13941 = T9 {"command"="", "data"=variant} ("element")
                n6472 = To Variant(anything=T3."mux10_1_channel7" ("mux10_1(x6)_encode")) -> (Variant=w13948:variant)
                n6473 = To Variant(anything=T2."mux6_1_channel5_3" ("mux6_1(3wires)_encode")) -> (Variant=w13946:variant)
                n6474 = To Variant(anything=T4."demux1_10_channel7" ("demux1_10(x6)_encode")) -> (Variant=w13942:variant)
                n6475 = To Variant(anything=bool[] [FALSE, FALSE, FALSE, FALSE, TRUE, FALSE]) -> (Variant=w13938:variant)
                n6476 = Bundle By Name(cluster=w13941, "command"="MEAS.AllRelaysOFF") -> (w13937:T9)
                n6477 = Bundle By Name(cluster=w13941, "command"="MEAS.mux10-1", "data"=w13948) -> (w13936:T9)
                n6478 = Bundle By Name(cluster=w13941, "command"="MEAS.mux6_1", "data"=w13946) -> (w13935:T9)
                n6479 = Bundle By Name(cluster=w13941, "command"="MEAS.demux1-10", "data"=w13942) -> (w13934:T9)
                n6480 = Bundle By Name(cluster=w13941, "command"="MEAS.eMIC", "data"=w13938) -> (w13933:T9)
                n6481 = Build Array(w13937, w13936, w13935, w13934, w13933) -> (w13918:T9[])
                n6482 = To Variant(anything=w13923) -> (Variant=w13921:variant)
                n6483 = To Variant(anything=w13923) -> (Variant=w13920:variant)
                n6484 = Bundle By Name(cluster=w13919, "command"="WaitFor") -> (w13917:T9)
                n6485 = Bundle By Name(cluster=w13919, "command"="MEAS.DMM dual read") -> (w13930:T9)
                n6486 = Bundle By Name(cluster=w13919, "command"="MEAS.requestAC", "data"=w13921) -> (w13929:T9)
                n6487 = Bundle By Name(cluster=w13919, "command"="Apps.WaitForEvent", "data"=w13920) -> (w13924:T9)
                n6488 = Bundle By Name(cluster=w13919, "command"="Apps.UI Update 1") -> (w13925:T9)
                n6489 = Build Array (concatenate)(w13918, w13917, w13930, w13929, w13924, w13925) -> (w13922:T9[])
              }
            }
          }
          frame True {
            n6490 = Bundle By Name(cluster=T9 {"command"="", "data"=variant} ("element"), "command"="Apps.UI Update 1") -> (w13952:T9)
            n6491 = Build Array(w13952) -> (w13951:T9[])
          }
        }
        n6492 = for {
          tunnel: w13867 -> [w13962] mode=indexing
          tunnel: w13875 -> [w13963]
          tunnel: [w13959] -> w13877 mode=indexing
          n6493 = Unbundle By Name(w13962) -> ("command"=w13961:string, "data"=w13960:variant)
          n6494 = call "App enquece.vi"("command data"=w13960, "command"=w13961, "queue in"=w13963) -> ("error out"=w13959:errorcluster)  [unwired: 7 in, 1 out]
        }
        n6495 = Merge Errors(w13878, w13877) -> (w13876:errorcluster)
      }
      frame "Test DRV 42A" {
        w13967 = 42 ("DUT index(0-59)")
        n6496 = disable-structure shown="LOGGING==TRUE" {
          disable-tunnel: w13972 -> [w14055 _]
          frame condition #0 (active) {
            n6497 = Empty String/Path?(string/path=w14055) -> (empty?=w14057:bool)
            n6498 = Select(t="Quece timeout", s=w14057, f=w14055) -> (s? t:f=w14054:string)
            n6499 = call "string log (SubVI).vi"("state Name"=w14054) -> ()  [unwired: 9 in, 2 out]
          }
          frame condition #1 {
          }
        }
        n6500 = Flush Queue(queue=w13973) -> (queue out=w13974:refnum<queue>)  [unwired: 1 in, 2 out]
        n6501 = Decrement(x=w13967) -> (x-1=w13971:i32)
        n6502 = Index Array(array=w13968, index=w13971) -> (element=w13969:refnum<vi>)
        n6503 = call "FGV DRV stand.vi"() -> ("Sub-Test.DCV"=w13964:bool)  [unwired: 10 in, 1 out]
        n6504 = call "FGV Driver Data.vi"("DUT index(1-60)"=w13967) -> ("DUT SC"=w13965:bool)  [unwired: 7 in, 3 out]
        n6505 = property class="ColBox"(reference=w13969, "Value"=u32 10000536 ("DRV 1")) -> ()  [unwired: 1 in, 2 out]
        n6506 = case shown="False" w13965 {
          tunnel: w13967 -> [w13985 _]
          tunnel: [w13984 w14050] -> w13966
          tunnel: w13964 -> [w13983 _]
          frame False {
            n6507 = case shown="True" w13983 {
              tunnel: w13985 -> [w13992 w14022]
              tunnel: [w14003 w14021] -> w13984
              frame False {
                w13989 = T9 {"command"="", "data"=variant} ("element")
                w14002 = T9 {"command"="", "data"=variant} ("element")
                n6508 = To Variant(anything=T3."mux10_1_channel7" ("mux10_1(x6)_encode")) -> (Variant=w14000:variant)
                n6509 = To Variant(anything=T4."demux1_10_channel7" ("demux1_10(x6)_encode")) -> (Variant=w13996:variant)
                n6510 = To Variant(anything=bool[] [FALSE, FALSE, FALSE, FALSE, FALSE, TRUE]) -> (Variant=w14011:variant)
                n6511 = Bundle By Name(cluster=w14002, "command"="MEAS.AllRelaysOFF") -> (w14010:T9)
                n6512 = Bundle By Name(cluster=w14002, "command"="MEAS.mux10-1", "data"=w14000) -> (w13993:T9)
                n6513 = Bundle By Name(cluster=w14002, "command"="MEAS.demux1-10", "data"=w13996) -> (w13994:T9)
                n6514 = Bundle By Name(cluster=w14002, "command"="MEAS.eMIC", "data"=w14011) -> (w13995:T9)
                n6515 = Build Array(w14010, w13993, w13994, w13995) -> (w13988:T9[])
                n6516 = To Variant(anything=w13992) -> (Variant=w13991:variant)
                n6517 = To Variant(anything=w13992) -> (Variant=w13990:variant)
                n6518 = Bundle By Name(cluster=w13989, "command"="MEAS.requestAC", "data"=w13991) -> (w14008:T9)
                n6519 = Bundle By Name(cluster=w13989, "command"="Apps.WaitForEvent", "data"=w13990) -> (w14004:T9)
                n6520 = Bundle By Name(cluster=w13989, "command"="Apps.UI Update 1") -> (w14005:T9)
                n6521 = Bundle By Name(cluster=w13989, "command"="WaitFor") -> (w13987:T9)
                n6522 = Build Array (concatenate)(w13988, w13987, w14008, w14004, w14005) -> (w14003:T9[])
              }
              frame True {
                w14018 = T9 {"command"="", "data"=variant} ("element")
                w14040 = T9 {"command"="", "data"=variant} ("element")
                n6523 = To Variant(anything=T3."mux10_1_channel7" ("mux10_1(x6)_encode")) -> (Variant=w14047:variant)
                n6524 = To Variant(anything=T2."mux6_1_channel6_3" ("mux6_1(3wires)_encode")) -> (Variant=w14045:variant)
                n6525 = To Variant(anything=T4."demux1_10_channel7" ("demux1_10(x6)_encode")) -> (Variant=w14041:variant)
                n6526 = To Variant(anything=bool[] [FALSE, FALSE, FALSE, FALSE, FALSE, TRUE]) -> (Variant=w14037:variant)
                n6527 = Bundle By Name(cluster=w14040, "command"="MEAS.AllRelaysOFF") -> (w14036:T9)
                n6528 = Bundle By Name(cluster=w14040, "command"="MEAS.mux10-1", "data"=w14047) -> (w14035:T9)
                n6529 = Bundle By Name(cluster=w14040, "command"="MEAS.mux6_1", "data"=w14045) -> (w14034:T9)
                n6530 = Bundle By Name(cluster=w14040, "command"="MEAS.demux1-10", "data"=w14041) -> (w14033:T9)
                n6531 = Bundle By Name(cluster=w14040, "command"="MEAS.eMIC", "data"=w14037) -> (w14032:T9)
                n6532 = Build Array(w14036, w14035, w14034, w14033, w14032) -> (w14017:T9[])
                n6533 = To Variant(anything=w14022) -> (Variant=w14020:variant)
                n6534 = To Variant(anything=w14022) -> (Variant=w14019:variant)
                n6535 = Bundle By Name(cluster=w14018, "command"="WaitFor") -> (w14016:T9)
                n6536 = Bundle By Name(cluster=w14018, "command"="MEAS.DMM dual read") -> (w14029:T9)
                n6537 = Bundle By Name(cluster=w14018, "command"="MEAS.requestAC", "data"=w14020) -> (w14028:T9)
                n6538 = Bundle By Name(cluster=w14018, "command"="Apps.WaitForEvent", "data"=w14019) -> (w14023:T9)
                n6539 = Bundle By Name(cluster=w14018, "command"="Apps.UI Update 1") -> (w14024:T9)
                n6540 = Build Array (concatenate)(w14017, w14016, w14029, w14028, w14023, w14024) -> (w14021:T9[])
              }
            }
          }
          frame True {
            n6541 = Bundle By Name(cluster=T9 {"command"="", "data"=variant} ("element"), "command"="Apps.UI Update 1") -> (w14051:T9)
            n6542 = Build Array(w14051) -> (w14050:T9[])
          }
        }
        n6543 = for {
          tunnel: w13966 -> [w14061] mode=indexing
          tunnel: w13974 -> [w14062]
          tunnel: [w14058] -> w13976 mode=indexing
